vi "Ion Sniffer.vi"() -> ()   [LabVIEW 2015]
uses:
  Type/_Source Type.ctl
  Type/_Log Command.ctl
  Type/_RT Command.ctl
  Type/_SaveOption.ctl
  Type/_RT Instrument State.ctl
  Type/_LC Command.ctl
  Configuration/_Global Configuration.vi
  <vilib>/Utility/config.llb/Read Key (Path).vi
  <vilib>/Utility/config.llb/Write Key (Path).vi
  <vilib>/Utility/config.llb/Read Key (String).vi
  <vilib>/Utility/config.llb/Write Key (String).vi
  LCDriver/_Global LC Driver.vi
  <vilib>/Utility/config.llb/Read Key (I32).vi
  <vilib>/Utility/config.llb/Write Key (I32).vi
  <vilib>/Utility/miscctls.llb/LVRectTypeDef.ctl
  <vilib>/Utility/config.llb/NI_LVConfig.lvlib
panel:
  out "RT Events":string
  out "Exhaust OK":bool
  out "CurGas OK":bool
  out "Pump OK":bool
  out "Interlock OK":bool
  out "Vac. Pressure:":sgl format="%#.2e"
  out "HSID Temp:":sgl
  out "Source 2 Temp:":sgl
  out "Source 2 Type:":T1 items=["None", "ESI", "APCI", "APPI", "MicroSpray"]
  out "Source 1 Temp:":sgl
  out "Source 1 Type:":T1 items=["None", "ESI", "APCI", "APPI", "MicroSpray"]
  in  "Display":bool
  in  "Acquisition":bool
  in  "Tuning":bool
  in  "Diagnostics":bool
  in  "Configuration":bool
  # "Source Status"
  # "Other Status"
  # "Torr"
  # "Interlocks:"
  # "Pump Speed:"
  # "Curtain Gas:"
  # "Exhaust Gas:"
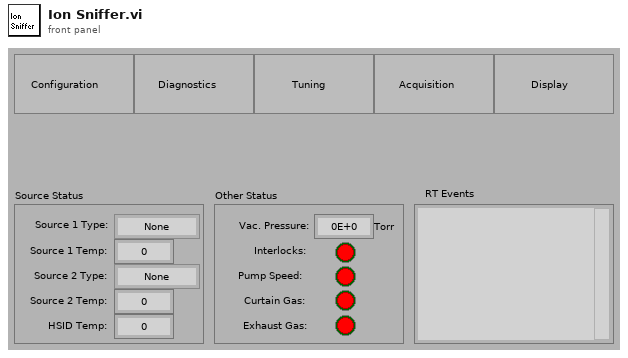
[diagram p1: front panel]
types:
  T1 = typedef "_Source Type.ctl" = i8
  T2 = typedef "_Log Command.ctl" = enum16{"No Command", "Open", "Read", "Write", "Close", "Check Size"}
  T3 = typedef "_RT Command.ctl" = enum16{"xml Start Run", "xml Start Actual Run", "xml Stop Run", "xml Runtime Update", "xml Get Status", "xml Get Table", "xml Set Table", "xml Get Configuration", "xml System Status", "xml Set LC Input Logic", "xml Get Data", "xml Get Info", "Start", "StartActualRun", "Stop", "Runtime Update", "Get Data", "Get Info", "Get Status", "Get Param", "Get Config", "Get Table", "Read ADC", "Set Oscillator", "Update Config", "Update Table", "Set All Pol", "Set Pol and DC", "Set Max Mass", "Toggle RP", "Toggle EL", "Set PIC", "Initialize Turbo", "Send Turbo Comm", "Close Turbo", "P1", "P2", "P3", "Send Serial", "Set LC Out", "Get LC In", "Read VAC", "Test Table", "Toggle Power", "Get Startup", "Set Startup", "Get ADC Table", "Set ADC Table", "Get Brief Status", "Get Detail Status", "Auxiliary Update", "Set CC Logics", "Set CC Input Logics", "Ignore Error", "invalid"}
  T4 = typedef "LVRectTypeDef.ctl" = cluster{"Left":i16, "Top":i16, "Right":i16, "Bottom":i16}
  T5 = typedef "_RT Instrument State.ctl" = enum16{"Initializing", "Mass Spectrometer is Off", "Starting Up", "Turning Power Off", "Going to Standby", "Roughing Pump Ready", "Turning Turbo Off", "Turbo Startup", "Turbopump Ready", "Checking Vacuum", "Going to Ready", "Ready", "Running", "Source Standby", "Lost Communication", "Shutting Down", "Fault", "24V Standby", "Go to 24V Standby", "Turbopump Ready-Waiting"}
  T6 = typedef "_SaveOption.ctl" = enum16{"Use Dialog", "Temporary File", "My Tables", "Full Path"}
  T7 = typedef "_LC Command.ctl" = enum16{"No Command", "Initialize", "Get Configuration", "Get Status", "Get LC Method Contents", "Oven OnOff", "Pump OnOFF", "Rinse Autosampler", "Run Sample", "Set EnvParameters", "Set Method", "Start Equilibration", "Stop Run", "Get LastError", "Clear Error", "Close"}
  T8 = typedef "NI_LVConfig.lvlib/Config Data RefNum.ctl" = refnum<k1>
  T9 = typedef "_LC Type.ctl" = enum16{"No LC", "Spark"}
  T10 = typedef "_RT Configuration 2.ctl" = cluster{"Name":string, "Ch#":u8, "Min":dbl, "Max":dbl, "Def+":dbl, "Def-":dbl, "Offset":dbl, "Slope":dbl, "Type":u8, "Description":string, "SettleT":dbl}
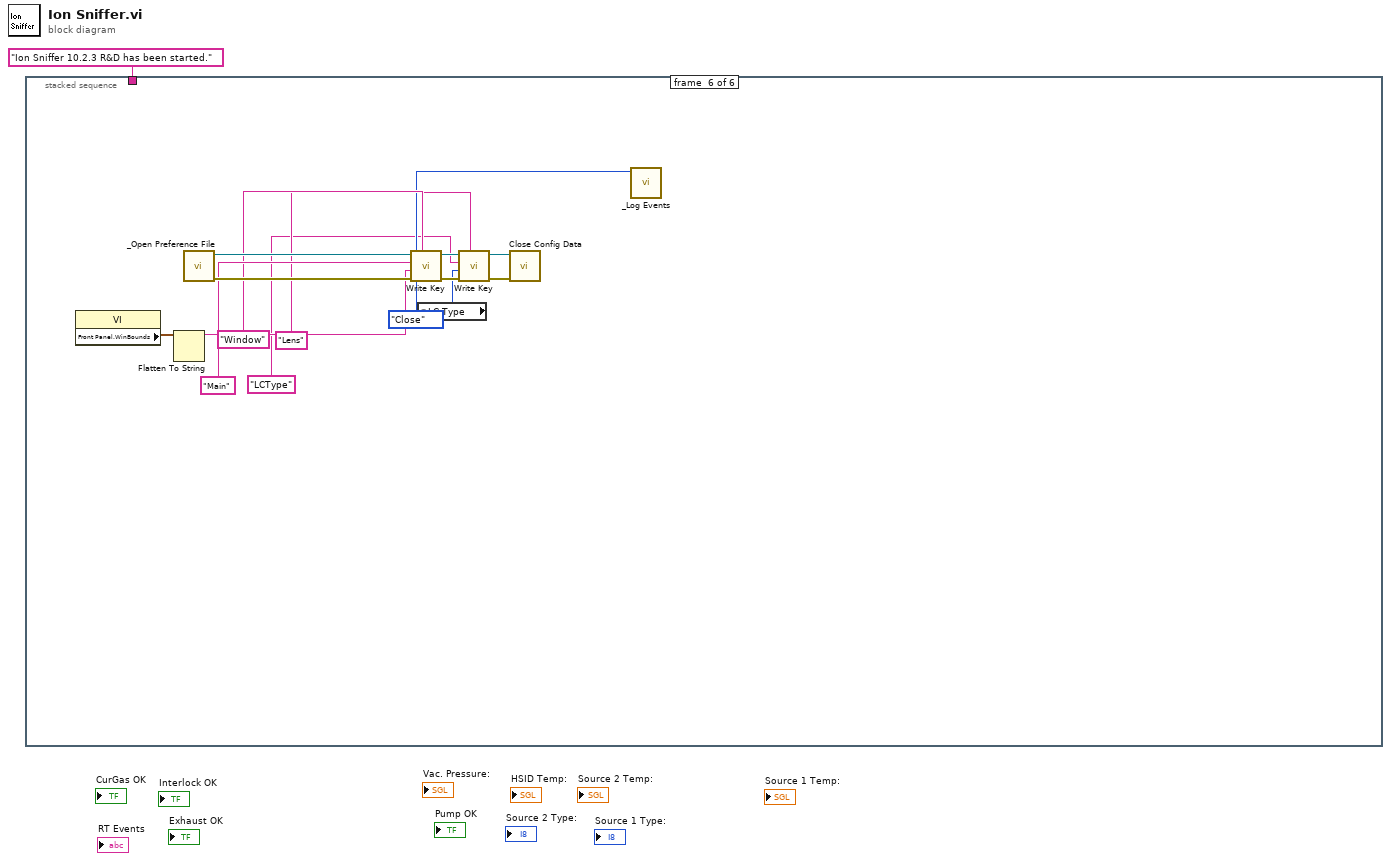
[diagram p0: block diagram]
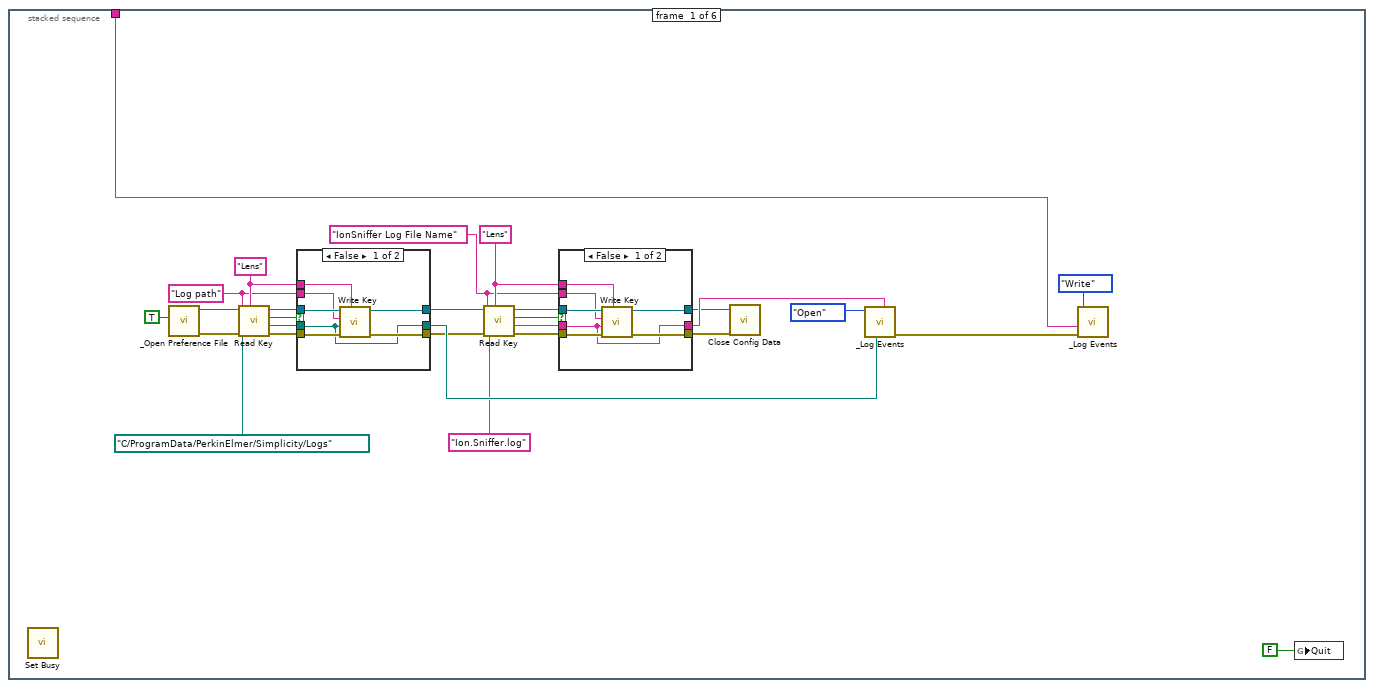
[diagram p2: hidden frame]
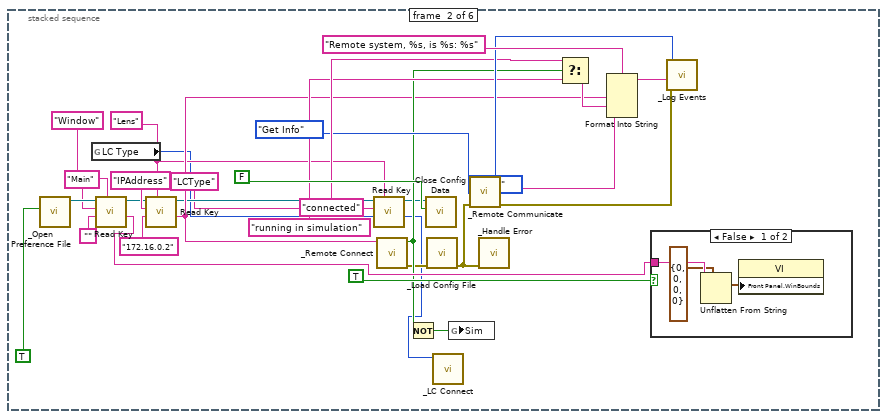
[diagram p5: hidden frame]
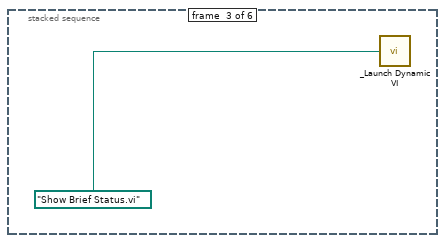
[diagram p7: hidden frame]
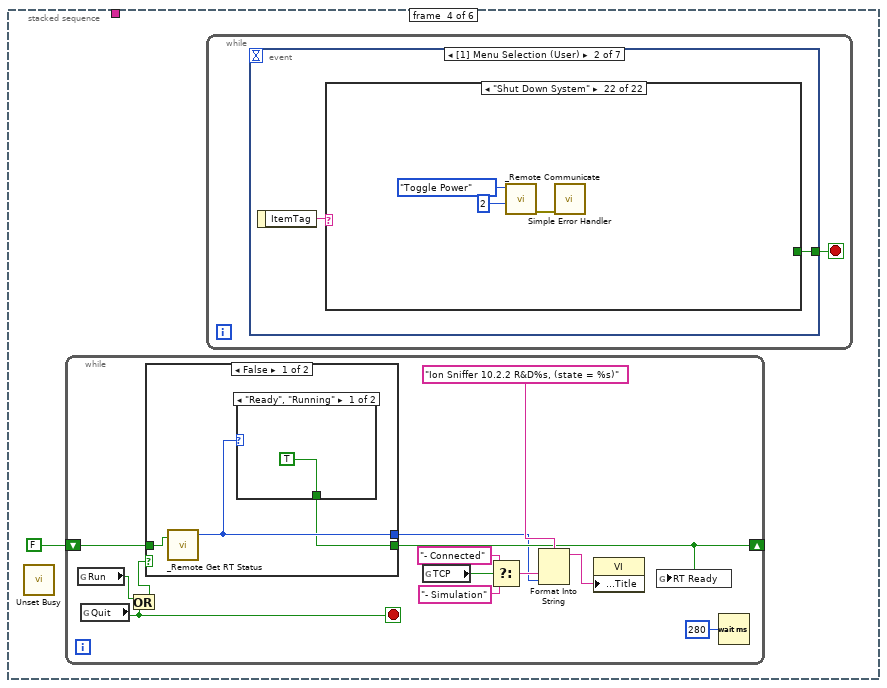
[diagram p8: hidden frame]
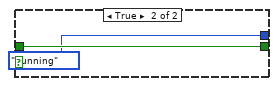
[diagram p10: hidden frame]
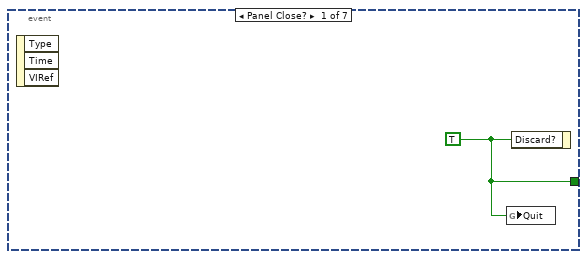
[diagram p11: hidden frame]
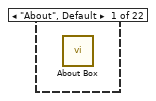
[diagram p12: hidden frame]
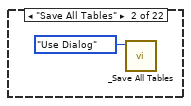
[diagram p13: hidden frame]
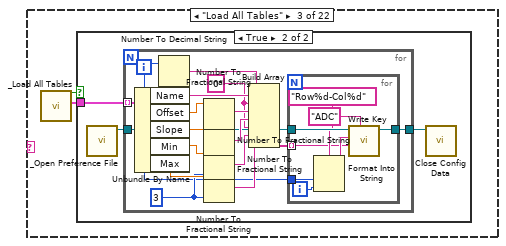
[diagram p14: hidden frame]
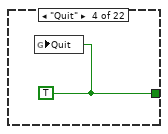
[diagram p16: hidden frame]
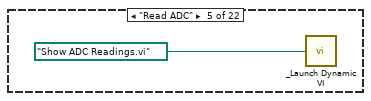
[diagram p17: hidden frame]
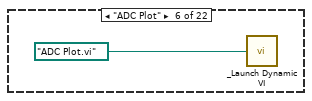
[diagram p18: hidden frame]
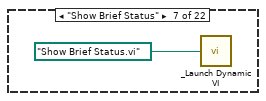
[diagram p19: hidden frame]
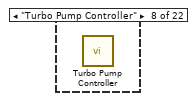
[diagram p20: hidden frame]
diagram:
  n1 = stacked-sequence {
    tunnel: "Ion Sniffer 10.2.3 R&D has been started." ("string") -> [w2 _ _ _ _ _]
    frame #0 {
      w6 = "IonSniffer Log File Name" ("key")
      w7 = "Lens" ("section")
      w12 = "Log path" ("key")
      w13 = "Lens" ("section")
      n2 = call <vilib>:"Set Busy.vi"() -> ()  [unwired: 4 in, 8 out]
      n3 = call "_Open Preference File.vi"("Initialize"=TRUE) -> ("error"=w21:errorcluster, "refnum"=w20:T8)  [unwired: 2 in, 3 out]
      n4 = call-poly <vilib>:"Read Key.vi"("section"=w13, "error in (no error)"=w21, "default value"=path "C:/ProgramData/PerkinElmer/Simplicity/Logs", "key"=w12, "refnum"=w20) -> ("error out"=w19:errorcluster, "value"=w17:path, "found?"=w18:bool, "refnum out"=w16:T8)  [unwired: 3 in]
      n5 = case shown="False" w18 {
        tunnel: w19 -> [w46 w49]
        tunnel: w17 -> [w40 w47]
        tunnel: w16 -> [w44 w48]
        tunnel: [w45 w49] -> w15
        tunnel: [w43 w48] -> w14
        tunnel: [w40 w47] -> w27
        tunnel: w13 -> [w42 _]
        tunnel: w12 -> [w41 _]
        frame False {
          n6 = call-poly <vilib>:"Write Key.vi"("section"=w42, "error in (no error)"=w46, "value"=w40, "key"=w41, "refnum"=w44) -> ("error out"=w45:errorcluster, "refnum out"=w43:T8)  [unwired: 4 in, 1 out]
        }
        frame True {
        }
      }
      n7 = call-poly <vilib>:"Read Key.vi"("section"=w7, "error in (no error)"=w15, "default value"="Ion.Sniffer.log", "key"=w6, "refnum"=w14) -> ("error out"=w8:errorcluster, "value"=w9:string, "found?"=w10:bool, "refnum out"=w11:T8)  [unwired: 3 in]
      n8 = case shown="False" w10 {
        tunnel: w8 -> [w36 w39]
        tunnel: w9 -> [w30 w37]
        tunnel: w11 -> [w34 w38]
        tunnel: [w35 w39] -> w4
        tunnel: [w33 w38] -> w5
        tunnel: [w30 w37] -> w28
        tunnel: w7 -> [w32 _]
        tunnel: w6 -> [w31 _]
        frame False {
          n9 = call-poly <vilib>:"Write Key.vi"("section"=w32, "error in (no error)"=w36, "value"=w30, "key"=w31, "refnum"=w34) -> ("error out"=w35:errorcluster, "refnum out"=w33:T8)  [unwired: 4 in, 1 out]
        }
        frame True {
        }
      }
      n10 = call <vilib>:"Close Config Data.vi"("error in (no error)"=w4, "refnum"=w5) -> ()  [unwired: 1 in, 9 out]
      n11 = call "_Log Events.vi"("File Name"=w28, "Log Path"=w27, "Log Command"=_Log_Command."Open" ("File Command")) -> ("error out"=w26:errorcluster)  [unwired: 5 in, 1 out]
      n12 = call "_Log Events.vi"("error in (no error)"=w26, "Event"=w2, "Log Command"=_Log_Command."Write" ("File Command")) -> ()  [unwired: 5 in, 2 out]
      n13 = global write "_Global Configuration.vi" "Quit"(FALSE ("Quit")) -> ()
    }
    frame #1 {
      w55 = "Lens" ("section")
      n14 = call "_Open Preference File.vi"("Initialize"=TRUE) -> ("refnum"=w75:T8)  [unwired: 2 in, 4 out]
      n15 = global read "_Global LC Driver.vi" "LC Type"() -> (w52:T9)
      n16 = call-poly <vilib>:"Read Key.vi"("section"="Window", "default value"="", "key"="Main" ("section"), "refnum"=w75) -> ("value"=w80:string, "refnum out"=w76:T8)  [unwired: 2 in, 4 out]
      n17 = call-poly <vilib>:"Read Key.vi"("section"=w55, "default value"="172.16.0.2", "key"="IPAddress" ("section"), "refnum"=w76) -> ("value"=w57:string, "refnum out"=w56:T8)  [unwired: 2 in, 4 out]
      n18 = call-poly <vilib>:"Read Key.vi"("section"=w55, "default value"=w52, "key"="LCType" ("section"), "refnum"=w56) -> ("value"=w51:i32, "refnum out"=w53:T8)  [unwired: 1 in, 5 out]
      n19 = call "_Remote Connect.vi"("IP Address"=w57) -> ("error out"=w60:errorcluster, "TCP"=w61:bool)  [unwired: 1 in, 4 out]
      n20 = Not(x=w61) -> (.not. x?=w62:bool)
      n21 = call <vilib>:"Close Config Data.vi"("write file if changed (T)"=FALSE ("write configuration file? (T)"), "refnum"=w53) -> ()  [unwired: 1 in, 9 out]
      n22 = call "_Load Config File.vi"("error in (no error)"=w60) -> ("error out"=w58:errorcluster)  [unwired: 6 out]
      n23 = call "_LC Connect.vi"("LC Type"=w51) -> ()  [unwired: 7 out]
      n24 = global write "_Global Configuration.vi" "Sim"(w62) -> ()
      n25 = call "_Remote Communicate.vi"("error in (no error)"=w58, "Command"=_RT_Command."Get Info") -> ("error out"=w59:errorcluster, "Info"=w63:string)  [unwired: 4 in, 2 out]
      n26 = call "_Handle Error.vi"("error in (no error)"=w58) -> ()  [unwired: 2 in, 5 out]
      n27 = Select(t="connected", s=w61, f="running in simulation") -> (s? t:f=w69:string)
      n28 = Format Into String(format string="Remote system, %s, is %s: %s", w57, w69, w63) -> (resulting string=w68:string)  [unwired: 2 in, 1 out]
      n29 = case shown="False" TRUE {
        tunnel: w80 -> [w83 _]
        frame False {
          n30 = Unflatten From String(type=T4 {"Left"=0, "Top"=0, "Right"=0, "Bottom"=0} ("Front Panel Window:Window Bounds"), binary string=w83) -> (value=w81:T4)  [unwired: 1 in, 4 out]
          n31 = property class="VI"("Front Panel.WinBounds"=w81) -> ()  [unwired: 2 in, 2 out]
        }
        frame True {
        }
      }
      n32 = call "_Log Events.vi"("error in (no error)"=w59, "Event"=w68, "Log Command"=_Log_Command."Write" ("File Command")) -> ()  [unwired: 5 in, 2 out]
    }
    frame #2 {
      n33 = call "_Launch Dynamic VI.vi"("VI Name"=path "Show Brief Status.vi" ("name or relative path")) -> ()  [unwired: 4 out]
    }
    frame #3 {
      n34 = call <vilib>:"Unset Busy.vi"() -> ()  [unwired: 2 in, 10 out]
      n35 = while {
        shift-right: [w90] -> _
        shift-left: FALSE -> [w98]
        stop <- w88 stop-if-true
        n36 = global read "_Global Configuration.vi" "Run"() -> (w87:bool)
        n37 = global read "_Global Configuration.vi" "Quit"() -> (w88:bool)
        n38 = Or(x=w87, y=w88) -> (x .or. y?=w86:bool)
        n39 = case shown="False" w86 {
          tunnel: w98 -> [w101 w104]
          tunnel: [w100 _RT_Instrument_State."Running" ("InstrState")] -> w89
          tunnel: [w99 w104] -> w90
          frame False {
            n40 = call "_Remote Get RT Status.vi"("RT Ready"=w101) -> ("InstrState"=w100:T5)  [unwired: 1 in, 2 out]
            n41 = case shown="\"Ready\", \"Running\"" w100 {
              tunnel: [TRUE _] -> w99
              frame "Ready", "Running" {
              }
              frame Default {
              }
            }
          }
          frame True {
          }
        }
        n42 = global read "_Global Configuration.vi" "TCP"() -> (w94:bool)
        n43 = Select(t="- Connected", s=w94, f="- Simulation") -> (s? t:f=w91:string)
        n44 = Format Into String(format string="Ion Sniffer 10.2.2 R&D%s, (state = %s)", w91, w89) -> (resulting string=w95:string)  [unwired: 2 in, 1 out]
        n45 = property class="VI"("Front Panel Window:Title"=w95) -> ()  [unwired: 2 in, 2 out]
        n46 = global write "_Global Configuration.vi" "RT Ready"(w90) -> ()
        n47 = Wait (ms)(milliseconds to wait=u32 280) -> ()  [unwired: 1 out]
      }
      n48 = while {
        stop <- w105 stop-if-true
        n49 = event shown="[1] Menu Selection (User)" {
          selector: _ -> [_ _ _ _ _ _ _]
          dyn-events: _ -> [_ _ _ _ _ _ _]
          timeout: _ -> [_ _ _ _ _ _ _]
          tunnel: [w106 w107 _ _ _ _ _] -> w105
          event Panel Close? {
            w106 = TRUE
            n50 = event-data() -> ()  [unwired: 4 out]
            n51 = global write "_Global Configuration.vi" "Quit"(w106) -> ()
            n52 = event-data("Discard?"=w106) -> ()  [unwired: 1 in, 1 out]
          }
          event Menu Selection (User) {
            n53 = event-data() -> ("ItemTag"=w108:string)  [unwired: 1 out]
            n54 = case shown="\"Shut Down System\"" w108 {
              tunnel: [_ _ _ w140 _ _ _ _ _ _ _ _ _ _ _ _ _ _ _ _ _ _] -> w107
              frame "About", Default {
                n55 = call "About Box.vi"() -> ()  [unwired: 1 out]
              }
              frame "Save All Tables" {
                n56 = call "_Save All Tables.vi"("SaveOption (Temporary File)"=_SaveOption."Use Dialog") -> ()  [unwired: 2 in, 5 out]
              }
              frame "Load All Tables" {
                n57 = call "_Load All Tables.vi"() -> ("ADC Table"=w110:T10[], "Loaded ADC"=w111:bool)  [unwired: 1 in, 5 out]
                n58 = case shown="True" w111 {
                  tunnel: w110 -> [_ w114]
                  frame False {
                  }
                  frame True {
                    n59 = call "_Open Preference File.vi"() -> ("refnum"=w113:T8)  [unwired: 3 in, 4 out]
                    n60 = for {
                      tunnel: w114 -> [w131] mode=indexing
                      tunnel: w113 -> [w118]
                      tunnel: [w116] -> w112
                      i -> [w117]
                      w121 = "0"
                      w126 = i16 3 ("precision (6)")
                      n61 = Unbundle By Name(w131) -> ("Name"=w124:string, "Offset"=w130:dbl, "Slope"=w129:dbl, "Min"=w128:dbl, "Max"=w127:dbl)
                      n62 = Number To Decimal String(number=w117) -> (decimal integer string=w125:string)  [unwired: 1 out]
                      n63 = Number To Fractional String(number=w130) -> (F-format string=w123:string)  [unwired: 3 out]
                      n64 = Number To Fractional String(number=w129) -> (F-format string=w122:string)  [unwired: 3 out]
                      n65 = Number To Fractional String(number=w128, precision (6)=w126) -> (F-format string=w120:string)  [unwired: 2 out]
                      n66 = Number To Fractional String(number=w127, precision (6)=w126) -> (F-format string=w119:string)  [unwired: 2 out]
                      n67 = Build Array(w125, w124, w121, w123, w122, w121, w120, w119) -> (w115:string[])
                      n68 = for {
                        tunnel: w118 -> [w139]
                        tunnel: [w138] -> w116
                        tunnel: w117 -> [w136]
                        tunnel: w115 -> [w132] mode=indexing
                        i -> [w137]
                        n69 = Format Into String(format string="Row%d-Col%d" ("section"), w136, w137) -> (resulting string=w134:string)  [unwired: 2 in, 1 out]
                        n70 = call-poly <vilib>:"Write Key.vi"("section"="ADC", "value"=w132, "key"=w134, "refnum"=w139) -> ("refnum out"=w138:T8)  [unwired: 2 in, 5 out]
                      }
                    }
                    n71 = call <vilib>:"Close Config Data.vi"("refnum"=w112) -> ()  [unwired: 2 in, 9 out]
                  }
                }
              }
              frame "Quit" {
                w140 = TRUE
                n72 = global write "_Global Configuration.vi" "Quit"(w140) -> ()
              }
              frame "Read ADC" {
                n73 = call "_Launch Dynamic VI.vi"("VI Name"=path "Show ADC Readings.vi" ("name or relative path")) -> ()  [unwired: 4 out]
              }
              frame "ADC Plot" {
                n74 = call "_Launch Dynamic VI.vi"("VI Name"=path "ADC Plot.vi" ("name or relative path")) -> ()  [unwired: 4 out]
              }
              frame "Show Brief Status" {
                n75 = call "_Launch Dynamic VI.vi"("VI Name"=path "Show Brief Status.vi" ("name or relative path")) -> ()  [unwired: 4 out]
              }
              frame "Turbo Pump Controller" {
                n76 = call "Turbo Pump Controller.vi"() -> ()  [unwired: 8 out]
              }
              frame "Leybold Pump Controller" {
                n77 = call "Turbo Pump Controller 2.vi"() -> ()  [unwired: 8 in]
              }
              frame "Syringe Pump Controller" {
                n78 = call "Syringe Pump Controller.vi"() -> ()  [unwired: 8 out]
              }
              frame "LCD Controller" {
                n79 = call "LCD Controller.vi"() -> ()  [unwired: 8 out]
              }
              frame "Start-Up Options" {
                n80 = call "Start Up Options.vi"() -> ()  [unwired: 1 in, 7 out]
              }
              frame "Source Controller" {
                n81 = call "Source Controller.vi"() -> ()  [unwired: 8 out]
              }
              frame "Serial Test Controller" {
                n82 = call "Serial Test Controller.vi"() -> ()  [unwired: 8 out]
              }
              frame "Read FPGA Map" {
                n83 = call "Show FPGA Map.vi"() -> ()  [unwired: 12 out]
              }
              frame "Test Table" {
                n84 = call "Table Test.vi"() -> ()  [unwired: 1 out]
              }
              frame "Re-Connect" {
                n85 = stacked-sequence {
                  tunnel: [_ w147 _] -> w144
                  frame #0 {
                    n86 = call <vilib>:"Set Busy.vi"() -> ()  [unwired: 4 in, 8 out]
                  }
                  frame #1 {
                    n87 = call "_Open Preference File.vi"() -> ("error"=w145:errorcluster, "refnum"=w146:T8)  [unwired: 3 in, 3 out]
                    n88 = call-poly <vilib>:"Read Key.vi"("section"="Lens", "error in (no error)"=w145, "default value"="172.16.0.2", "key"="IPAddress" ("section"), "refnum"=w146) -> ("error out"=w151:errorcluster, "value"=w149:string, "refnum out"=w152:T8)  [unwired: 1 in, 3 out]
                    n89 = call <vilib>:"Close Config Data.vi"("error in (no error)"=w151, "write file if changed (T)"=FALSE ("write configuration file? (T)"), "refnum"=w152) -> ()  [unwired: 9 out]
                    n90 = call "_Remote Connect.vi"("IP Address"=w149) -> ("error out"=w148:errorcluster)  [unwired: 1 in, 5 out]
                    n91 = call "_Load Config File.vi"("error in (no error)"=w148) -> ("error out"=w147:errorcluster)  [unwired: 6 out]
                  }
                  frame #2 {
                    n92 = call <vilib>:"Unset Busy.vi"() -> ()  [unwired: 2 in, 10 out]
                  }
                }
                n93 = call "_Handle Error.vi"("error in (no error)"=w144) -> ()  [unwired: 2 in, 5 out]
              }
              frame "mzData Converter" {
                n94 = call "_mzData Converter.vi"() -> ()  [unwired: 2 out]
              }
              frame "txtData Converter" {
                n95 = call "_txtData Converter.vi"() -> ()  [unwired: 2 out]
              }
              frame "Start System" {
                n96 = call "_Remote Communicate.vi"("DC Param"=u16 0, "Command"=_RT_Command."Toggle Power") -> ("error out"=w156:errorcluster)  [unwired: 4 in, 3 out]
                n97 = call <vilib>:"Simple Error Handler.vi"("error in (no error)"=w156) -> ()  [unwired: 1 in, 8 out]
              }
              frame "Goto Roughing Pump On Standby" {
                n98 = call "_Remote Communicate.vi"("DC Param"=u16 1, "Command"=_RT_Command."Toggle Power") -> ("error out"=w159:errorcluster)  [unwired: 4 in, 3 out]
                n99 = call <vilib>:"Simple Error Handler.vi"("error in (no error)"=w159) -> ()  [unwired: 1 in, 8 out]
              }
              frame "Shut Down System" {
                n100 = call "_Remote Communicate.vi"("DC Param"=u16 2, "Command"=_RT_Command."Toggle Power") -> ("error out"=w162:errorcluster)  [unwired: 4 in, 3 out]
                n101 = call <vilib>:"Simple Error Handler.vi"("error in (no error)"=w162) -> ()  [unwired: 1 in, 8 out]
              }
            }
          }
          event "Configuration": Value Change {
            n102 = event-data() -> ()  [unwired: 7 out]
            n103 = call "Edit Configuration.vi"() -> ()  [unwired: 8 out]
          }
          event "Diagnostics": Value Change {
            n104 = event-data() -> ()  [unwired: 7 out]
            n105 = call "Diagnostic.vi"() -> ()  [unwired: 8 out]
          }
          event "Tuning": Value Change {
            n106 = event-data() -> ()  [unwired: 7 out]
            n107 = global read "_Global Configuration.vi" "RT Ready"() -> (w165:bool)
            n108 = case shown="True" w165 {
              frame False {
                n109 = One Button Dialog(message="System is not ready.") -> ()  [unwired: 2 out]
              }
              frame True {
                n110 = call "Tuning.vi"() -> ()  [unwired: 8 out]
              }
            }
          }
          event "Acquisition": Value Change {
            n111 = event-data() -> ()  [unwired: 7 out]
            n112 = global read "_Global Configuration.vi" "RT Ready"() -> (w167:bool)
            n113 = case shown="False" w167 {
              frame False {
                n114 = One Button Dialog(message="System is not ready.") -> ()  [unwired: 2 out]
              }
              frame True {
                n115 = call "Acquisition.vi"() -> ()  [unwired: 8 out]
              }
            }
          }
          event "Display": Value Change {
            n116 = event-data() -> ()  [unwired: 7 out]
            n117 = call "Data Viewer.vi"() -> ()  [unwired: 1 in]
          }
        }
      }
    }
    frame #4 {
      n118 = call "_LC Send Command.vi"("Command"=_LC_Command."Close") -> ()  [unwired: 9 in, 2 out]
      n119 = call "_Remote Communicate.vi"("DC Param"=u16 1, "Command"=_RT_Command."Ignore Error") -> ()  [unwired: 4 in, 4 out]
    }
    frame #5 {
      n120 = property class="VI"() -> ("Front Panel.WinBounds"=w181:T4)  [unwired: 2 in, 2 out]
      n121 = Flatten To String(anything=w181) -> (data string=w180:string)  [unwired: 1 in, 4 out]
      n122 = call "_Open Preference File.vi"() -> ("error"=w184:errorcluster, "refnum"=w185:T8)  [unwired: 3 in, 3 out]
      n123 = call-poly <vilib>:"Write Key.vi"("section"="Window", "error in (no error)"=w184, "value"=w180, "key"="Main" ("section"), "refnum"=w185) -> ("error out"=w178:errorcluster, "refnum out"=w177:T8)  [unwired: 1 in, 4 out]
      n124 = global read "_Global LC Driver.vi" "LC Type"() -> (w174:T9)
      n125 = call-poly <vilib>:"Write Key.vi"("section"="Lens", "error in (no error)"=w178, "value"=w174, "key"="LCType" ("section"), "refnum"=w177) -> ("error out"=w172:errorcluster, "refnum out"=w173:T8)  [unwired: 5 out]
      n126 = call <vilib>:"Close Config Data.vi"("error in (no error)"=w172, "refnum"=w173) -> ()  [unwired: 1 in, 9 out]
      n127 = call "_Log Events.vi"("Log Command"=_Log_Command."Close" ("File Command")) -> ()  [unwired: 7 in, 2 out]
    }
  }
